vi "Get X Array dx.vi"(8 "error in (no error)":errorcluster, 11 "XY-data":cluster{"X-array":dbl[], "Y-array":dbl[]}) -> (0 "error out":errorcluster, 1 "X0":dbl, 2 "dX":dbl, 3 "XY-data out":cluster{"X-array":dbl[], "Y-array":dbl[]})   [LabVIEW 2016, in "xy_utilities.lvlib"]
uses:
  xy_utilities.lvlib
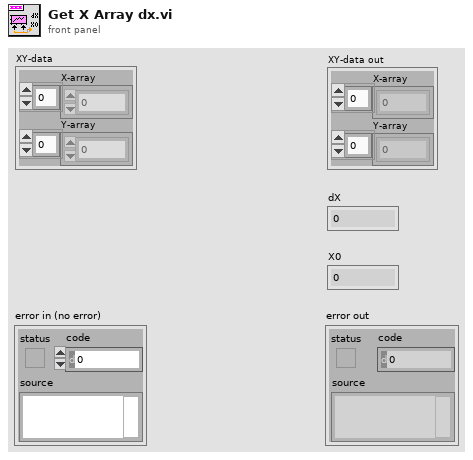
[diagram p1: front panel]
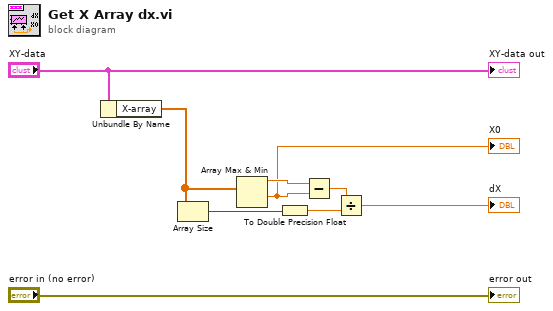
[diagram p0: block diagram]
diagram:
  n1 = Unbundle By Name("XY-data") -> ("X-array"=w2:dbl[])
  n2 = Array Size(array=w2) -> (size(s)=w7:i32)
  n3 = Array Max & Min(array=w2) -> (max value=w9:dbl, min value=w5:dbl)  [unwired: 2 out]
  "X0" <- w5
  n4 = To Double Precision Float(number=w7) -> (double precision float=w6:dbl)
  n5 = Subtract(x=w9, y=w5) -> (x-y=w8:dbl)
  n6 = Divide(x=w8, y=w6) -> (x/y=→"dX":dbl)
  "error out" <- "error in (no error)"
  "XY-data out" <- "XY-data"
